vi "email_.vi"(0 "vent":bool, 1 "clim":bool, 8 "mode":string, 9 "humid":string, 10 "temp":string, 11 "to":string="dhiadridi06@gmail.com") -> (3 "error out":errorcluster)   [LabVIEW 2021]
uses:
  <vilib>/smtpClient/Set Message Text.vi
  <vilib>/smtpClient/LabVIEWSMTPClient.lvlib
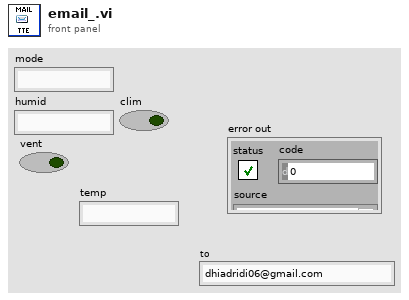
[diagram p1: front panel]
types:
  T1 = typedef "LabVIEWSMTPClient.lvlib/SmtpClientHandle.ctl" = refnum<k1>
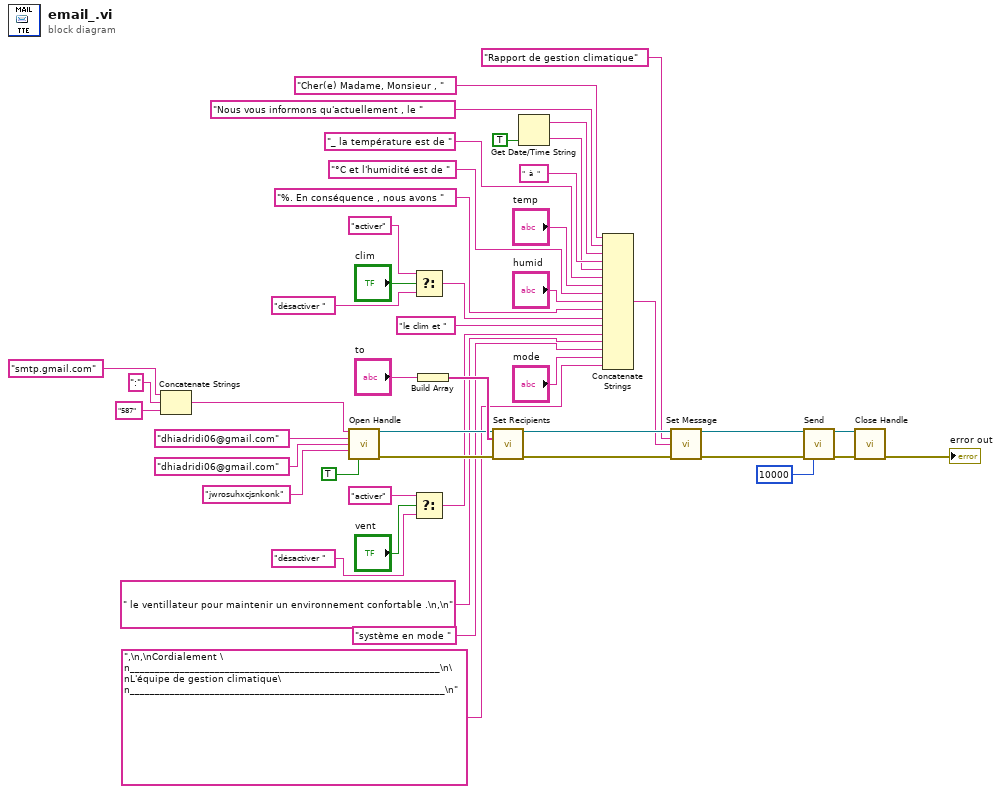
[diagram p0: block diagram]
diagram:
  n1 = Concatenate Strings "Concatenate Strings"("smtp.gmail.com" ("string"), ":" ("string"), "587" ("string")) -> (w45:string)
  n2 = call <vilib>:"Open Handle.vi"("server address"=w45, "from"="dhiadridi06@gmail.com", "username"="dhiadridi06@gmail.com", "password"="jwrosuhxcjsnkonk", "use TLS (false)"=TRUE) -> ("handle out"=w36:T1, "error out"=w37:errorcluster)  [unwired: 9 in]
  n3 = Select(t="activer", s="clim", f="désactiver ") -> (s? t:f=w9:string)
  n4 = Select(t="activer", s="vent", f="désactiver ") -> (s? t:f=w7:string)
  n5 = Build Array("to") -> (w44:string[])
  n6 = call <vilib>:"Set Recipients.vi"("handle in"=w36, "to"=w44, "error in (no error)"=w37) -> ("handle out"=w42:T1, "error out"=w43:errorcluster)  [unwired: 11 in]
  n7 = Get Date/Time String(want seconds? (F)=TRUE) -> (date string=w25:string, time string=w23:string)  [unwired: 2 in]
  n8 = Concatenate Strings("Cher(e) Madame, Monsieur , " ("string"), "Nous vous informons qu'actuellement , le " ("string"), w25, "  à  " ("string"), w23, "_ la température est de " ("string"), "temp", "°C et l'humidité est de " ("string"), "humid", "%. En conséquence , nous avons " ("string"), w9, "le clim et " ("string"), w7, " le ventillateur pour maintenir un environnement confortable .\n,\n" ("string"), "système en mode " ("string"), "mode", ",\n,\nCordialement \n______________________________________________________________\n\nL'équipe de gestion climatique\n_______________________________________________________________\n" ("string")) -> (w21:string)
  n9 = call-poly <vilib>:"Set Message.vi"("handle in"=w42, "subject"="Rapport de gestion climatique", "plain text message"=w21, "error in (no error)"=w43) -> ("handle out"=w40:T1, "error out"=w41:errorcluster)  [unwired: 10 in]
  n10 = call <vilib>:"Send.vi"("handle in"=w40, "error in (no error)"=w41, "timeout in ms (10000)"=10000) -> ("handle out"=w38:T1, "error out"=w39:errorcluster)  [unwired: 10 in, 1 out]
  n11 = call <vilib>:"Close Handle.vi"("handle in"=w38, "error in (no error)"=w39) -> ("error out"=→"error out":errorcluster)  [unwired: 12 in, 1 out]
